vi "Write VI Data File.vi"(8 "error in":errorcluster, 11 "Path":path) -> (0 "error out":errorcluster, 3 "saved file":path=path "C:/")   [LabVIEW 2016]
doc: "Drop this VI into any VI will save a copy of the data on the front panel as a VI without a diagram."
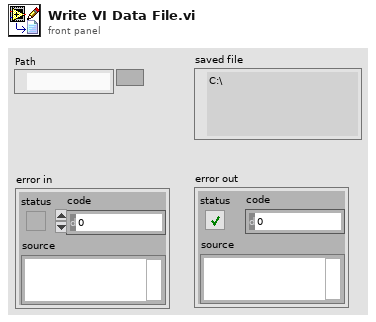
[diagram p1: front panel]
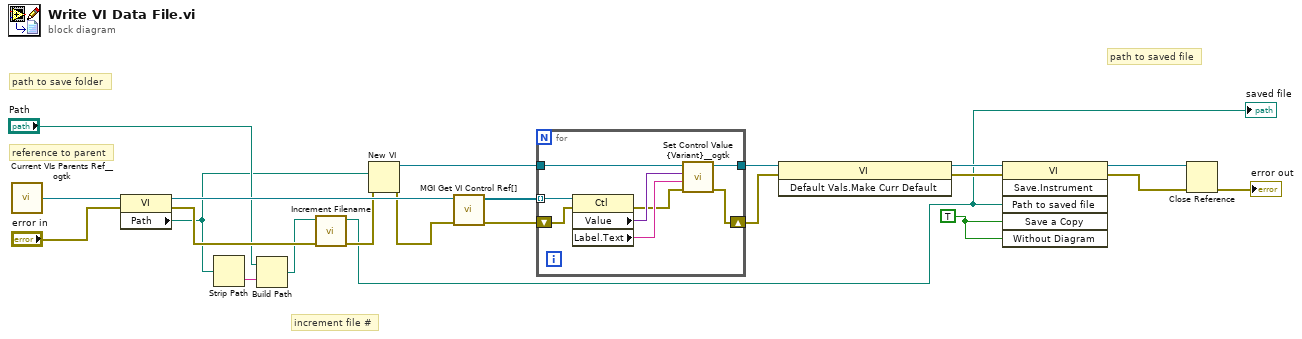
[diagram p0: block diagram]
diagram:
  w2 = TRUE ("Without Diagram")
  # "path to saved file"
  # "increment file #"
  # "path to save folder"
  # "reference to parent"
  n1 = call "Current VIs Parents Ref__ogtk.vi"() -> ("Calling VI's Reference"=w7:refnum<vi>)  [unwired: 2 in]
  n2 = property class="VI"(reference=w7, error in="error in") -> (reference out=w11:refnum<vi>, error out=w12:errorcluster, "Path"=w5:path)
  n3 = Strip Path(path=w5) -> (name=w3:string)  [unwired: 1 out]
  n4 = Build Path(base path="Path", name or relative path=w3) -> (appended path=w4:path)
  n5 = call "Increment Filename.vi"("error in (no error)"=w12, "Path"=w4) -> ("error out"=w9:errorcluster, "Modified Path"=w1:path)  [unwired: 8 in]
  "saved file" <- w1
  n6 = New VI(8:w9, 10:w5) -> (0:w8:errorcluster, 3:w10:refnum<vi>)  [unwired: 5 in]
  n7 = call "MGI Get VI Control Ref[].vi"("error in"=w8, "VI (Caller)"=w11) -> ("error out"=w18:errorcluster, "Control[i]"=w22:refnum<vi>[])  [unwired: 6 in, 2 out]
  n8 = for {
    tunnel: w22 -> [w30] mode=indexing
    shift-right: [w23] -> w17
    shift-left: w18 -> [w25]
    tunnel: w10 -> [w27]
    tunnel: [w26] -> w15
    n9 = property class="Ctl"(reference=w30, error in=w25) -> (error out=w24:errorcluster, "Value"=w29:variant, "Label.Text"=w28:string)  [unwired: 1 out]
    n10 = call "Set Control Value {Variant}__ogtk.vi"("error in (no error)"=w24, "Control Name (\"\": use variant name)"=w28, "Value"=w29, "VI Refnum"=w27) -> ("error out"=w23:errorcluster, "VI Refnum dup"=w26:refnum<vi>)  [unwired: 6 in]
  }
  n11 = invoke class="VI" method="Default Vals.Make Curr Default"(reference=w15, error in=w17) -> (reference out=w21:refnum<vi>, error out=w19:errorcluster)  [unwired: 1 in, 1 out]
  n12 = invoke class="VI" method="Save.Instrument"(reference=w21, error in=w19, "Path to saved file"=w1, "Save a Copy"=w2, "Without Diagram"=w2) -> (reference out=w20:refnum<vi>, error out=w14:errorcluster)  [unwired: 1 in, 4 out]
  n13 = Close Reference(reference=w20, error in (no error)=w14) -> (error out=→"error out":errorcluster)
